vi "Copy String.vi"(8 "error in":errorcluster, 9 "free (F)":bool, 10 "size":i32, 11 "pointer":i64) -> (0 "error out":errorcluster, 3 "string":string)   [LabVIEW 2020, in "G-Unicode.lvlib"]
doc: "Copy a string pointed to by <b>pointer</b> from a library into LabVIEW. The <b>size</b> is the number of bytes to be copied.\n\nSet <b>free</b> to True to free memory allocated by malloc(). Only set this if you know the allocated memory isn't being reused, or is free'd elsewhere."
uses:
  G-Unicode.lvlib
  4d47babd-4a2d-4eb7-b91b-7e707d692665.vi
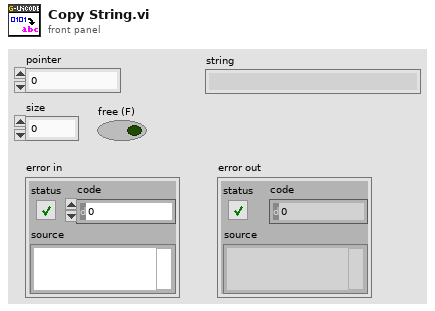
[diagram p1: front panel]
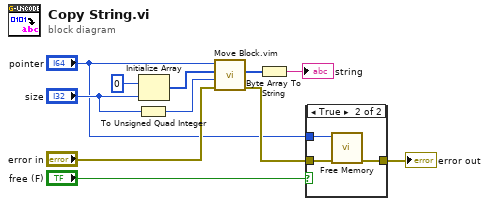
[diagram p0: block diagram]
diagram:
  n1 = To Unsigned Quad Integer(1:"size") -> (0:w8:u64)
  n2 = Initialize Array(u8 0, "size") -> (w9:u8[])
  n3 = call "Move Block.vim"("error in"="error in", "memory size"=w8, "memory"=w9, "pointer"="pointer") -> ("error out"=w4:errorcluster, "filled memory"=w11:u8[])  [unwired: 6 in]
  n4 = Byte Array To String(unsigned byte array=w11) -> (string=→"string":string)
  n5 = case shown="True" "free (F)" {
    tunnel: w4 -> [w12 w15]
    tunnel: [w12 w14] -> w3
    tunnel: "pointer" -> [_ w13]
    frame False {
    }
    frame True {
      n6 = call "Free Memory.vi"("error in"=w15, "pointer"=w13) -> ("error out"=w14:errorcluster)  [unwired: 9 in]
    }
  }
  "error out" <- w3
